vi "gfitsio-read-image-subset-i16-scalar.vi"(4 "npixels (rest)":i32[](array[numeric]), 6 "fpixel (origin)":i32[](array[numeric]), 7 "inc (1)":i32[](array[numeric]), 8 "error in (no error)":errorcluster, 11 "gfits refnum":T1) -> (0 "error out":errorcluster, 2 "data":u8, 3 "dup gfits refnum":T1)   [LabVIEW 2019, in "gfitsio.lvlib"]
doc: "Read a rectangular subset of the FITS data array. <B>fpixel</B>, <b>npixels</b>, and <b>inc</b> must have the same number of elements as the image has dimensions. <b>fpixel</b> specifies the first pixel in the subset. <b>npixels</b> specifies the number of pixels to read along each image dimension, and should be at least 1 for each dimension. The number of elements greater than 1 in <b>npixels</b> determines the dimensionality of the resulting array, and should match the dimensions of the array returned by the particular instance of the polymorphic GFITSIO read function used. <b>inc</b> specifies the decimation to use along each dimension of the image. 2 will read every other pixel, 3 will read every third pixel, and so on. <B>fpixel</B>, <b>npixels</b>, and <b>inc</b> must be specified in ROW-MAJOR order, with the fastest changing dimension (NAXIS1) listed last and the slowest changing dimension listed first. The array that is returned will be structured according to <B>npixels</B>."
uses:
  gfitsio.lvlib
  gfitsio-refnum.ctl
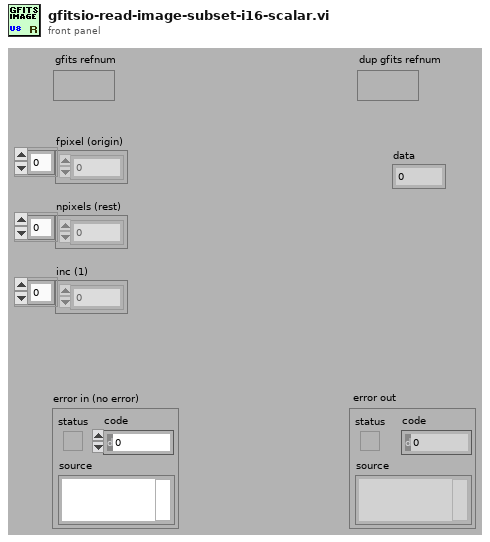
[diagram p1: front panel]
types:
  T1 = typedef "gfitsio.lvlib/gfitsio-refnum.ctl" = refnum<k1>
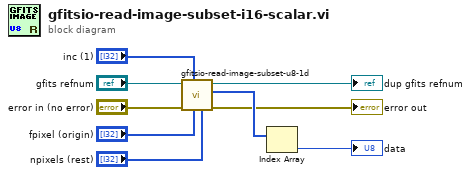
[diagram p0: block diagram]
diagram:
  n1 = call "gfitsio-read-image-subset-u8-1d.vi"("npixels (rest)"="npixels (rest)", "fpixel (origin)"="fpixel (origin)", "inc (1)"="inc (1)", "error in (no error)"="error in (no error)", "gfits refnum"="gfits refnum") -> ("error out"=→"error out":errorcluster, "data"=w6:u8[], "dup gfits refnum"=→"dup gfits refnum":T1)  [unwired: 4 in]
  n2 = Index Array(array=w6) -> (element=→"data":u8)  [unwired: 1 in]
